vi "midiOutPlayer.Core.vi"(7 "notifier out":refnum<notifier>, 10 "MIDI Events":T1(array[cluster]), 11 "midi out":refnum<class "midi.lvclass">) -> ()   [LabVIEW 2020, in "midi.lvclass"]
uses:
  midi.lvclass
  midi.lvclass/midi.ctl
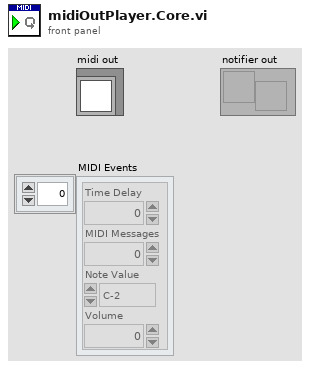
[diagram p1: front panel]
types:
  T1 = cluster{"Time Delay":u32, "MIDI Messages":u16, "Note Value":enum8{"C-2", "C#-2", "D-2", "D#-2", "E-2", "F-2", "F#-2", "G-2", "G#-2", "A-2", "A#-2", "B-2", "C-1", "C#-1", "D-1", "D#-1", "E-1", "F-1", "F#-1", "G-1", "G#-1", "A-1", "A#-1", "B-1", "C0", "C#0", "D0", "D#0", "E0", "F0", "F#0", "G0", "G#0", "A0", "A#0", "B0", "C1", "C#1", "D1", "D#1", "E1", "F1", "F#1", "G1", "G#1", "A1", "A#1", "B1", "C2", "C#2", "D2", "D#2", "E2", "F2", "F#2", "G2", "G#2", "A2", "A#2", "B2", "C3", "C#3", "D3", "D#3", "E3", "F3", "F#3", "G3", "G#3", "A3", "A#3", "B3", "C4", "C#4", "D4", "D#4", "E4", "F4", "F#4", "G4", "G#4", "A4", "A#4", "B4", "C5", "C#5", "D5", "D#5", "E5", "F5", "F#5", "G5", "G#5", "A5", "A#5", "B5", "C6", "C#6", "D6", "D#6", "E6", "F6", "F#6", "G6", "G#6", "A6", "A#6", "B6", "C7", "C#7", "D7", "D#7", "E7", "F7", "F#7", "G7", "G#7", "A7", "A#7", "B7", "C8", "C#8", "D8", "D#8", "E8", "F8", "F#8", "G"}, "Volume":u8}[]
  T2 = map{enum8{"C-2", "C#-2", "D-2", "D#-2", "E-2", "F-2", "F#-2", "G-2", "G#-2", "A-2", "A#-2", "B-2", "C-1", "C#-1", "D-1", "D#-1", "E-1", "F-1", "F#-1", "G-1", "G#-1", "A-1", "A#-1", "B-1", "C0", "C#0", "D0", "D#0", "E0", "F0", "F#0", "G0", "G#0", "A0", "A#0", "B0", "C1", "C#1", "D1", "D#1", "E1", "F1", "F#1", "G1", "G#1", "A1", "A#1", "B1", "C2", "C#2", "D2", "D#2", "E2", "F2", "F#2", "G2", "G#2", "A2", "A#2", "B2", "C3", "C#3", "D3", "D#3", "E3", "F3", "F#3", "G3", "G#3", "A3", "A#3", "B3", "C4", "C#4", "D4", "D#4", "E4", "F4", "F#4", "G4", "G#4", "A4", "A#4", "B4", "C5", "C#5", "D5", "D#5", "E5", "F5", "F#5", "G5", "G#5", "A5", "A#5", "B5", "C6", "C#6", "D6", "D#6", "E6", "F6", "F#6", "G6", "G#6", "A6", "A#6", "B6", "C7", "C#7", "D7", "D#7", "E7", "F7", "F#7", "G7", "G#7", "A7", "A#7", "B7", "C8", "C#8", "D8", "D#8", "E8", "F8", "F#8", "G"}, cluster{"Time Delay":u32, "MIDI Messages":u16, "Note Value":enum8{"C-2", "C#-2", "D-2", "D#-2", "E-2", "F-2", "F#-2", "G-2", "G#-2", "A-2", "A#-2", "B-2", "C-1", "C#-1", "D-1", "D#-1", "E-1", "F-1", "F#-1", "G-1", "G#-1", "A-1", "A#-1", "B-1", "C0", "C#0", "D0", "D#0", "E0", "F0", "F#0", "G0", "G#0", "A0", "A#0", "B0", "C1", "C#1", "D1", "D#1", "E1", "F1", "F#1", "G1", "G#1", "A1", "A#1", "B1", "C2", "C#2", "D2", "D#2", "E2", "F2", "F#2", "G2", "G#2", "A2", "A#2", "B2", "C3", "C#3", "D3", "D#3", "E3", "F3", "F#3", "G3", "G#3", "A3", "A#3", "B3", "C4", "C#4", "D4", "D#4", "E4", "F4", "F#4", "G4", "G#4", "A4", "A#4", "B4", "C5", "C#5", "D5", "D#5", "E5", "F5", "F#5", "G5", "G#5", "A5", "A#5", "B5", "C6", "C#6", "D6", "D#6", "E6", "F6", "F#6", "G6", "G#6", "A6", "A#6", "B6", "C7", "C#7", "D7", "D#7", "E7", "F7", "F#7", "G7", "G#7", "A7", "A#7", "B7", "C8", "C#8", "D8", "D#8", "E8", "F8", "F#8", "G"}, "Volume":u8}}
  T3 = cluster{"Time Delay":u32, "MIDI Messages":u16, "Note Value":enum8{"C-2", "C#-2", "D-2", "D#-2", "E-2", "F-2", "F#-2", "G-2", "G#-2", "A-2", "A#-2", "B-2", "C-1", "C#-1", "D-1", "D#-1", "E-1", "F-1", "F#-1", "G-1", "G#-1", "A-1", "A#-1", "B-1", "C0", "C#0", "D0", "D#0", "E0", "F0", "F#0", "G0", "G#0", "A0", "A#0", "B0", "C1", "C#1", "D1", "D#1", "E1", "F1", "F#1", "G1", "G#1", "A1", "A#1", "B1", "C2", "C#2", "D2", "D#2", "E2", "F2", "F#2", "G2", "G#2", "A2", "A#2", "B2", "C3", "C#3", "D3", "D#3", "E3", "F3", "F#3", "G3", "G#3", "A3", "A#3", "B3", "C4", "C#4", "D4", "D#4", "E4", "F4", "F#4", "G4", "G#4", "A4", "A#4", "B4", "C5", "C#5", "D5", "D#5", "E5", "F5", "F#5", "G5", "G#5", "A5", "A#5", "B5", "C6", "C#6", "D6", "D#6", "E6", "F6", "F#6", "G6", "G#6", "A6", "A#6", "B6", "C7", "C#7", "D7", "D#7", "E7", "F7", "F#7", "G7", "G#7", "A7", "A#7", "B7", "C8", "C#8", "D8", "D#8", "E8", "F8", "F#8", "G"}, "Volume":u8}
  T4 = enum8{"C-2", "C#-2", "D-2", "D#-2", "E-2", "F-2", "F#-2", "G-2", "G#-2", "A-2", "A#-2", "B-2", "C-1", "C#-1", "D-1", "D#-1", "E-1", "F-1", "F#-1", "G-1", "G#-1", "A-1", "A#-1", "B-1", "C0", "C#0", "D0", "D#0", "E0", "F0", "F#0", "G0", "G#0", "A0", "A#0", "B0", "C1", "C#1", "D1", "D#1", "E1", "F1", "F#1", "G1", "G#1", "A1", "A#1", "B1", "C2", "C#2", "D2", "D#2", "E2", "F2", "F#2", "G2", "G#2", "A2", "A#2", "B2", "C3", "C#3", "D3", "D#3", "E3", "F3", "F#3", "G3", "G#3", "A3", "A#3", "B3", "C4", "C#4", "D4", "D#4", "E4", "F4", "F#4", "G4", "G#4", "A4", "A#4", "B4", "C5", "C#5", "D5", "D#5", "E5", "F5", "F#5", "G5", "G#5", "A5", "A#5", "B5", "C6", "C#6", "D6", "D#6", "E6", "F6", "F#6", "G6", "G#6", "A6", "A#6", "B6", "C7", "C#7", "D7", "D#7", "E7", "F7", "F#7", "G7", "G#7", "A7", "A#7", "B7", "C8", "C#8", "D8", "D#8", "E8", "F8", "F#8", "G"}
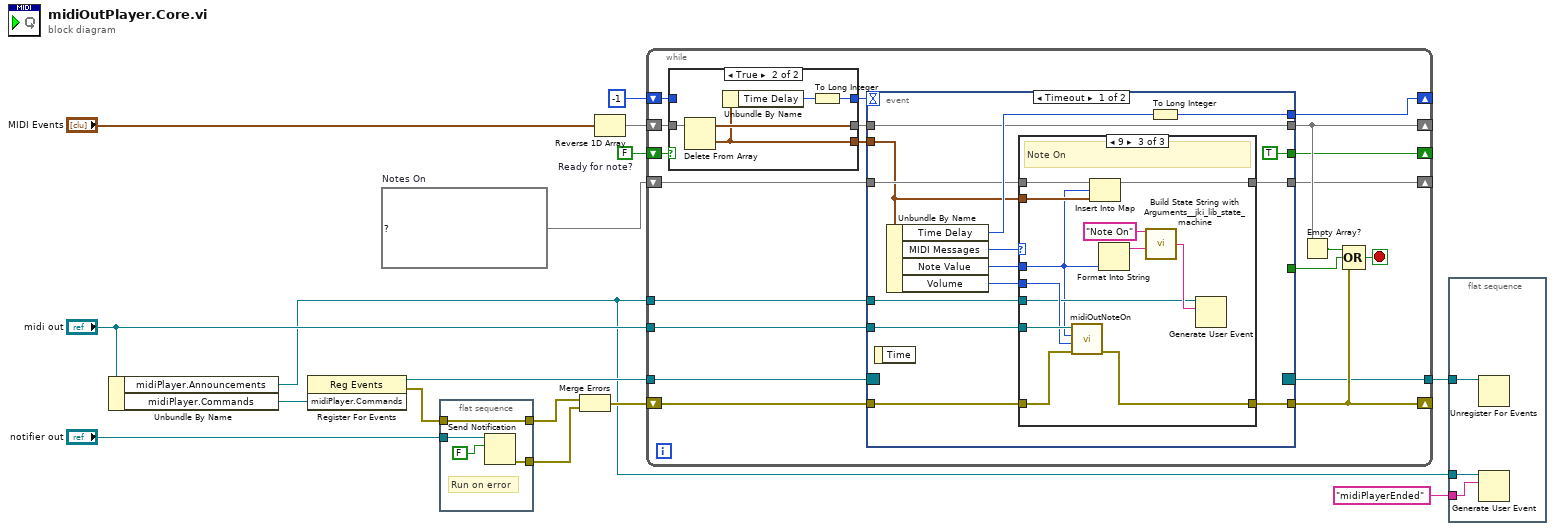
[diagram p0: block diagram]
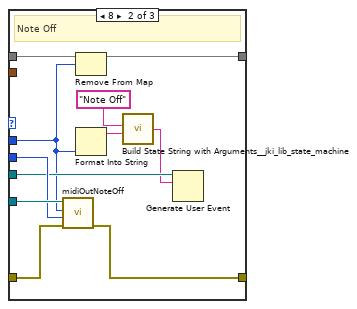
[diagram p4: hidden frame]
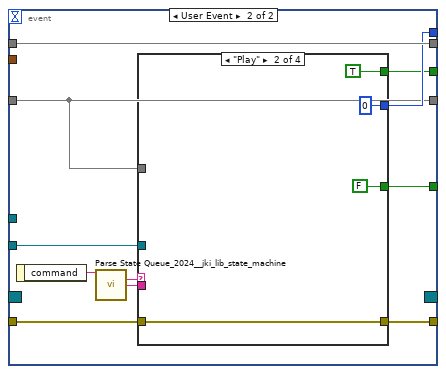
[diagram p5: hidden frame]
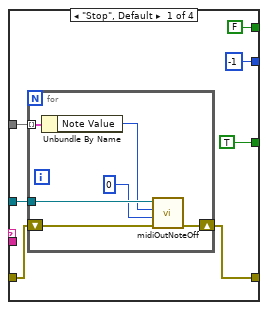
[diagram p6: hidden frame]
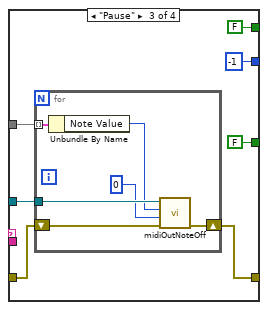
[diagram p7: hidden frame]
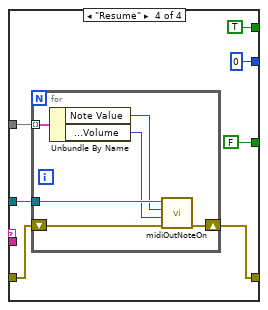
[diagram p8: hidden frame]
diagram:
  w1 = FALSE  # Ready for note?
  w2 = T2 {}  # Notes On
  n1 = Unbundle By Name("midi out") -> ("midiPlayer.Announcements"=w3:refnum<user-event>, "midiPlayer.Commands"=w4:refnum<user-event>)
  n2 = register-events(w4) -> (reference out=w8:refnum<event-registration>, error out=w9:errorcluster)  [unwired: 2 in]
  n3 = flat-sequence {
    tunnel: "notifier out" -> [w20]
    tunnel: [w18] -> w11
    tunnel: [w17] -> w10
    tunnel: w9 -> [w17]
    frame #0 {
      # "Run on error"
      n4 = Send Notification(notification=FALSE, notifier=w20) -> (error out=w18:errorcluster)  [unwired: 1 in, 1 out]
    }
  }
  n5 = Merge Errors(w10, w11) -> (w7:errorcluster)
  n6 = Reverse 1D Array(array="MIDI Events") -> (reversed array=w16:T1)
  n7 = while {
    shift-right: [w38] -> _
    shift-left: w16 -> [w27]
    shift-right: [w36] -> _
    shift-left: w7 -> [w40]
    shift-right: [w39] -> _
    shift-left: -1 -> [w22]
    tunnel: [w34] -> w13
    tunnel: w8 -> [w33]
    tunnel: "midi out" -> [w32]
    tunnel: w3 -> [w30]
    shift-right: [w28] -> _
    shift-left: w2 -> [w29]
    shift-right: [w21] -> _
    shift-left: w1 -> [w23]
    stop <- w35 stop-if-true
    n8 = case shown="True" w23 {
      tunnel: w27 -> [w41 w47]
      tunnel: [w41 w46] -> w26
      tunnel: [_ w43] -> w25
      tunnel: [w42 w44] -> w24
      tunnel: w22 -> [w42 _]
      frame False {
      }
      frame True {
        n9 = Delete From Array(array=w47) -> (deleted portion=w43:T3, array with subset deleted=w46:T1)  [unwired: 2 in]
        n10 = Unbundle By Name(w43) -> ("Time Delay"=w45:u32)
        n11 = To Long Integer(number=w45) -> (32bit integer=w44:i32)
      }
    }
    n12 = event shown="[0] Timeout" {
      selector: w33 -> [_ _]
      dyn-events: [_ _] -> w34
      timeout: w24 -> [_ _]
      tunnel: w32 -> [w60 w88]
      tunnel: w40 -> [w57 w95]
      tunnel: w26 -> [w50 w97]
      tunnel: [w50 w97] -> w38
      tunnel: [w56 w96] -> w36
      tunnel: [w54 w93] -> w39
      tunnel: [_ w94] -> w31
      tunnel: w30 -> [w48 _]
      tunnel: w29 -> [w53 w89]
      tunnel: [w52 w89] -> w28
      tunnel: w25 -> [w51 _]
      tunnel: [TRUE w87] -> w21
      event Timeout {
        n13 = event-data() -> ()  [unwired: 1 in, 1 out]
        n14 = Unbundle By Name(w51) -> ("Time Delay"=w55:u32, "MIDI Messages"=w61:u16, "Note Value"=w59:T4, "Volume"=w58:u8)
        n15 = case shown="9" w61 {
          tunnel: w60 -> [_ w74 w86]
          tunnel: w59 -> [_ w67 w76]
          tunnel: w58 -> [_ w73 w85]
          tunnel: w57 -> [w63 w72 w84]
          tunnel: [w63 w71 w83] -> w56
          tunnel: w53 -> [w62 w70 w82]
          tunnel: w51 -> [_ _ w81]
          tunnel: [w62 w69 w80] -> w52
          tunnel: w48 -> [_ w68 w77]
          frame 0, Default {
          }
          frame 8 {
            # "Note Off"
            n16 = call "midiOutNoteOff.vi"("error in"=w72, "Velocity (0-127)"=w73, "Note (0-127)"=w67, "midi in"=w74) -> ("error out"=w71:errorcluster)  [unwired: 6 in, 1 out]
            n17 = Remove From Map(10:w67, 11:w70) -> (3:w69:T2)  [unwired: 2 out]
            n18 = Format Into String(w67) -> (resulting string=w66:string)  [unwired: 3 in, 1 out]
            n19 = call <vilib>:"Build State String with Arguments__jki_lib_state_machine.vi"("Arguments (\"\")"=w66, "State"="Note Off") -> ("State with Arguments"=w64:string)  [unwired: 4 in]
            n20 = Generate User Event(user event=w68, event data cluster=w64) -> ()  [unwired: 2 in, 2 out]
          }
          frame 9 {
            # "Note On"
            n21 = call "midiOutNoteOn.vi"("error in"=w84, "Velocity (0-127)"=w85, "Note (0-127)"=w76, "midi in"=w86) -> ("error out"=w83:errorcluster)  [unwired: 6 in, 1 out]
            n22 = Insert Into Map(map in=w82, key=w76, value=w81) -> (map out=w80:T2)  [unwired: 2 out]
            n23 = Format Into String(w76) -> (resulting string=w79:string)  [unwired: 3 in, 1 out]
            n24 = call <vilib>:"Build State String with Arguments__jki_lib_state_machine.vi"("Arguments (\"\")"=w79, "State"="Note On") -> ("State with Arguments"=w78:string)  [unwired: 4 in]
            n25 = Generate User Event(user event=w77, event data cluster=w78) -> ()  [unwired: 2 in, 2 out]
          }
        }
        n26 = To Long Integer(number=w55) -> (32bit integer=w54:i32)
      }
      event User Event {
        n27 = event-data() -> ("command"=w92:string)  [unwired: 1 in]
        n28 = call <vilib>:"Parse State Queue_2024__jki_lib_state_machine.vi"("State Queue"=w92) -> ("Current State"=w91:string, "Arguments"=w90:string)  [unwired: 12 in, 1 out]
        n29 = case shown="\"Play\"" w91 {
          tunnel: [w100 w113 w116 w129] -> w96
          tunnel: w95 -> [w101 w113 w117 w130]
          tunnel: [TRUE FALSE FALSE FALSE] -> w94
          tunnel: [-1 0 -1 0] -> w93
          tunnel: w90 -> [_ _ _ _]
          tunnel: w89 -> [w102 _ w118 w131]
          tunnel: w88 -> [w99 _ w119 w132]
          tunnel: [FALSE TRUE FALSE TRUE] -> w87
          frame "Stop", Default {
            n30 = for {
              tunnel: w99 -> [w110]
              tunnel: w102 -> [w109] mode=indexing
              shift-right: [w105] -> w100
              shift-left: w101 -> [w106]
              n31 = Unbundle By Name(w109) -> ("Note Value"=w108:T4)
              n32 = call "midiOutNoteOff.vi"("error in"=w106, "Velocity (0-127)"=0, "Note (0-127)"=w108, "midi in"=w110) -> ("error out"=w105:errorcluster)  [unwired: 6 in, 1 out]
            }
          }
          frame "Play" {
          }
          frame "Pause" {
            n33 = for {
              tunnel: w119 -> [w127]
              tunnel: w118 -> [w126] mode=indexing
              shift-right: [w122] -> w116
              shift-left: w117 -> [w123]
              n34 = Unbundle By Name(w126) -> ("Note Value"=w125:T4)
              n35 = call "midiOutNoteOff.vi"("error in"=w123, "Velocity (0-127)"=0, "Note (0-127)"=w125, "midi in"=w127) -> ("error out"=w122:errorcluster)  [unwired: 6 in, 1 out]
            }
          }
          frame "Resume" {
            n36 = for {
              tunnel: w132 -> [w139]
              tunnel: w131 -> [w140] mode=indexing
              shift-right: [w135] -> w129
              shift-left: w130 -> [w136]
              n37 = Unbundle By Name(w140) -> ("Note Value"=w138:T4, "Note Attributes.Volume"=w137:u8)
              n38 = call "midiOutNoteOn.vi"("error in"=w136, "Velocity (0-127)"=w137, "Note (0-127)"=w138, "midi in"=w139) -> ("error out"=w135:errorcluster)  [unwired: 6 in, 1 out]
            }
          }
        }
      }
    }
    n39 = Empty Array?(array=w38) -> (empty?=w37:bool)
    n40 = Compound Arithmetic op=OR(w37, w31, w36) -> (w35:bool)
  }
  n41 = flat-sequence {
    tunnel: w13 -> [w143]
    tunnel: w3 -> [w142]
    tunnel: "midiPlayerEnded" ("event data") -> [w141]
    frame #0 {
      n42 = Unregister For Events(event registration refnum=w143) -> ()  [unwired: 1 in, 1 out]
      n43 = Generate User Event(user event=w142, event data cluster=w141) -> ()  [unwired: 2 in, 2 out]
    }
  }
